vi "Get Greeter_req.vi"(8 "error in (no error)":errorcluster, 11 "gRPCid":T1) -> (0 "error out":errorcluster, 2 "package_templatemessage":T2, 3 "gRPCid out":T1)   [LabVIEW 2019, in "Generated_server.lvlib"]
uses:
  Generated_server.lvlib
  Greeter_req.ctl
  Greeter_req_req_oneof/Greeter_req_req_oneof.lvclass
  Greeter_MessageA.ctl
  <vilib>/gRPC/LabVIEW gRPC Library/Shared/grpcId.ctl
  Greeter_req_Flat.ctl
  Greeter_MessageA_Flat.ctl
  Greeter_req_req_oneof/Greeter_req_req_oneof.lvclass/Greeter_req_req_oneof.ctl
  2ed25e12-861d-4677-8ead-ace2906b2041.vi
  <vilib>/gRPC/LabVIEW gRPC Library/Shared/TranslateGrpcError.vi
  FlatToRichGreeter_MessageA.vi
  Greeter_req_req_oneof/Setreq_id.vi
  Greeter_req_req_oneof/Setreq_name.vi
  <vilib>/gRPC/LabVIEW gRPC Library/Server API/Server/Get Server DLL Path.vi
  <vilib>/Utility/error.llb/Error Cluster From Error Code.vi
  <vilib>/Utility/error.llb/Simple Error Handler.vi
  Greeter_req_req_oneof/GetFieldFromProtobufIndexGreeter_req_req_oneof.vi
  <vilib>/gRPC/LabVIEW gRPC Library/grpc-lvsupport-release.lvlib
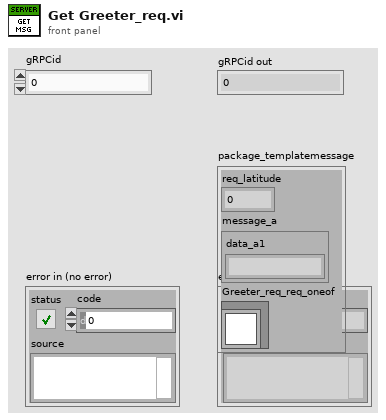
[diagram p1: front panel]
types:
  T1 = typedef "grpc-lvsupport-release.lvlib/grpcId.ctl" = u64
  T2 = typedef "Generated_server.lvlib/Greeter_req.ctl" = cluster{"req_latitude":i32, "message_a":T3, "Greeter_req_req_oneof":refnum<class "Greeter_req_req_oneof.lvclass">}
  T3 = typedef "Generated_server.lvlib/Greeter_MessageA.ctl" = cluster{"data_a1":string}
  T4 = typedef "Generated_server.lvlib/Greeter_req_Flat.ctl" = cluster{"req_latitude":i32, "message_a":T5, "Greeter_req_req_oneof_selected_index":i32, "req_id":i32, "req_name":string}
  T5 = typedef "Generated_server.lvlib/Greeter_MessageA_Flat.ctl" = cluster{"data_a1":string}
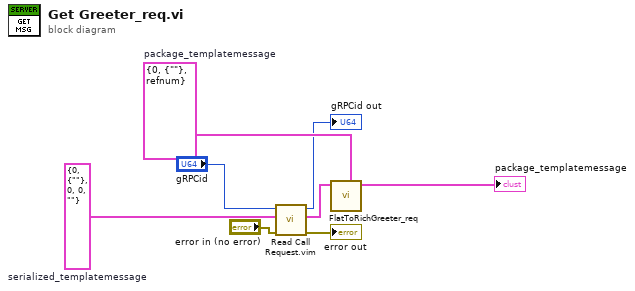
[diagram p0: block diagram]
diagram:
  w6 = T4 {"req_latitude"=0, "message_a"={"data_a1"=""}, "Greeter_req_req_oneof_selected_index"=0, "req_id"=0, "req_name"=""}  # serialized_templatemessage
  w5 = T2 {"req_latitude"=0, "message_a"={"data_a1"=""}, "Greeter_req_req_oneof"=refnum}  # package_templatemessage
  n1 = call "Read Call Request.vim"("error in"="error in (no error)", "Request Type"=w6, "gRPCid in"="gRPCid") -> ("error out"=→"error out":errorcluster, "Request Data"=w4:T4, "gRPCid out"=→"gRPCid out":T1)  [unwired: 6 in]
  n2 = call "FlatToRichGreeter_req.vi"("OutputClusterType"=w5, "InputCluster"=w4) -> ("OutputCluster"=→"package_templatemessage":T2)  [unwired: 9 in]
